vi "reset FPGA DO.vi"() -> ()   [LabVIEW 2012]
doc: "SciScan 1.2 160622"
uses:
  Custom Controls/biotfile select.ctl
  GFG/GFGstringGet.vi
  <vilib>/FPGAPlugInAG/PXIe-7962R/niLvFpga_Open_PXIe-7962R.vi
  <vilib>/rvi/interface/common/dynamic/niFpgaDynamicAddResources.vi
  <vilib>/FPGAPlugInAG/PXIe-7961R/niLvFpga_Open_PXIe-7961R.vi
  <vilib>/FPGAPlugInAG/Dynamic/niLvFpga_Run_Dynamic.vi
  <vilib>/FPGAPlugInAG/Dynamic/niLvFpga_Abort_Dynamic.vi
  <vilib>/FPGAPlugInAG/Dynamic/niLvFpga_Close_Dynamic.vi
  <vilib>/rvi/interface/nirviOpenFPGA/nirviOpenFPGA.xnode
  fpga bitfiles/bak/7962with5751_resetDO.lvbitx
  fpga bitfiles/bak/7961with5734_resetDO.lvbitx
  fpga bitfiles/7962with5734_resetDO.lvbitx
  <vilib>/rvi/interface/nirviMethod/nirviMethod.xnode
  <vilib>/rvi/interface/nirviCloseFPGA/nirviCloseFPGA.xnode
  GFG/GFG library.lvlib
panel:
  out "error out":errorcluster
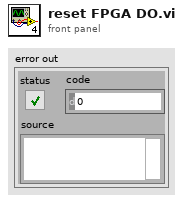
[diagram p1: front panel]
types:
  T1 = typedef "biotfile select.ctl" = enum16{"7962with5751_512px_40Mhz", "7962with5751_512px_50Mhz", "7961with5734_1024px_120Mhz or ext lasersync", "7962with5734_1024px_120Mhz or ext lasersync", "7962with5734_512px_120Mhz or ext lasersync", "7961with5734_512px_120Mhz or ext lasersync", "7962with5751_12kHz_512px_50MHz_4ch", "7962with5751_1536px_2ch_40Mhz", "7962with5751_1536px_2ch_50Mhz", "7962with5751_12kHz_1024px_2ch_50MHz"}
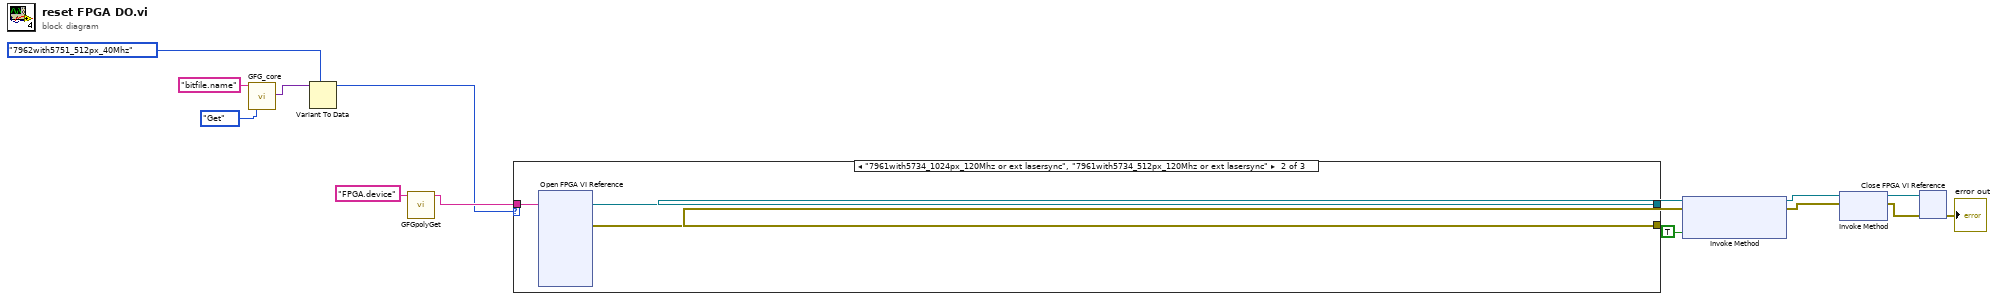
[diagram p0: block diagram]
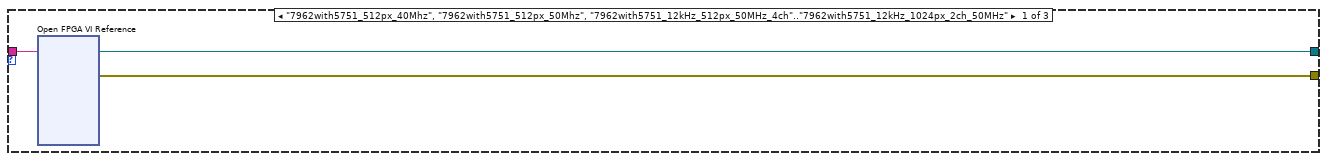
[diagram p2: hidden frame]
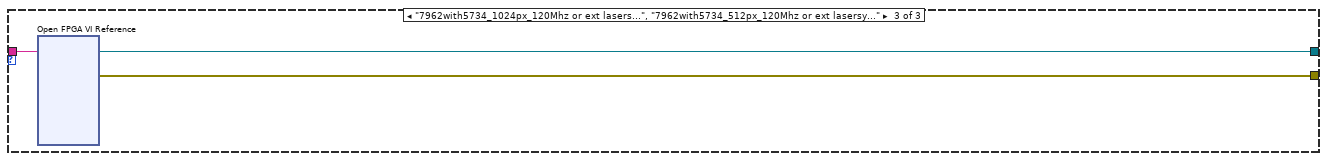
[diagram p3: hidden frame]
diagram:
  n1 = call "GFG_core.vi"("Variable Name in"="bitfile.name", "Action"=enum16{"Init", "Set", "Get", "Clear"}."Get") -> ("Variant Out"=w11:variant)  [unwired: 11 in, 6 out]
  n2 = Variant To Data(type=biotfile_select."7962with5751_512px_40Mhz" ("bitfile name"), Variant=w11) -> (data=w2:T1)  [unwired: 1 in, 1 out]
  n3 = call-poly "GFGpolyGet.vi"("Variable Name in"="FPGA.device") -> ("String"=w14:string)  [unwired: 9 in, 1 out]
  n4 = case shown="\"7961with5734_1024px_120Mhz or ext lasersync\", \"7961with5734_512px_120Mhz or ext lasersync\"" w2 {
    tunnel: [w18 w21 w24] -> w10
    tunnel: w14 -> [w17 w20 w23]
    tunnel: [w16 w19 w22] -> w8
    frame "7962with5751_512px_40Mhz", "7962with5751_512px_50Mhz", "7962with5751_12kHz_512px_50MHz_4ch".."7962with5751_12kHz_1024px_2ch_50MHz" {
      n5 = xnode "Open FPGA VI Reference"("resource name"=w17) -> ("FPGA VI Reference Out"=w18:refnum<k20>, "error out"=w16:errorcluster)  [unwired: 1 in]
    }
    frame "7961with5734_1024px_120Mhz or ext lasersync", "7961with5734_512px_120Mhz or ext lasersync" {
      n6 = xnode "Open FPGA VI Reference"("resource name"=w20) -> ("FPGA VI Reference Out"=w21:refnum<k20>, "error out"=w19:errorcluster)  [unwired: 1 in]
    }
    frame "7962with5734_1024px_120Mhz or ext lasersync", "7962with5734_512px_120Mhz or ext lasersync" {
      n7 = xnode "Open FPGA VI Reference"("resource name"=w23) -> ("FPGA VI Reference Out"=w24:refnum<k20>, "error out"=w22:errorcluster)  [unwired: 1 in]
    }
  }
  n8 = xnode "Invoke Method"("FPGA VI Reference In"=w10, "error in"=w8, "Wait Until Done (F)"=TRUE) -> ("FPGA VI Reference Out"=w7:refnum<k20>, "error out"=w5:errorcluster)
  n9 = xnode "Invoke Method"("FPGA VI Reference In"=w7, "error in"=w5) -> ("FPGA VI Reference Out"=w6:refnum<k20>, "error out"=w4:errorcluster)
  n10 = xnode "Close FPGA VI Reference"("FPGA VI Reference In"=w6, "error in"=w4) -> ("error out"=→"error out":errorcluster)
